vi "EXPT_IMGCAP.vi"(0 "Refnums":T1, 1 "Number of wavelengths":u16(ring) items=["1", "2", "3", "4", "5", "6"], 5 "Saved positions":dbl[][](array[numeric]), 9 "Filter array":dbl[](array[numeric]), 11 "Error in":errorcluster, 12 "Img data":refnum<queue>, 13 "State queue cam":refnum<queue>) -> (4 "Avg intensity":T2(array[cluster]), 6 "Number of positions":i32, 8 "XYZpos":cluster{dbl, dbl, dbl}, 15 "error out":errorcluster)   [LabVIEW 2018]
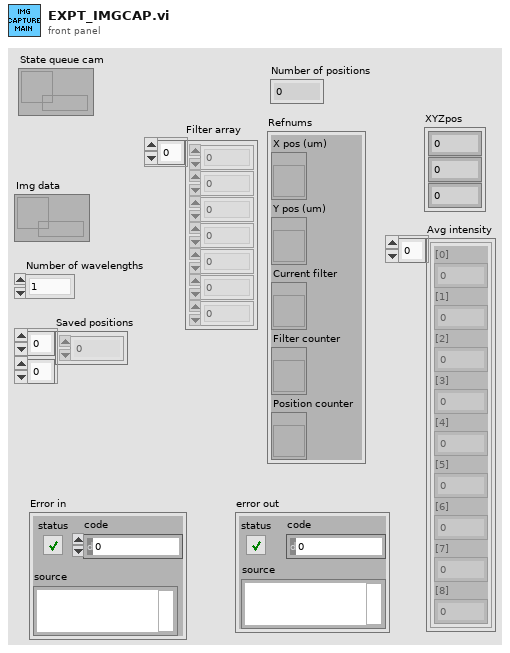
[diagram p1: front panel]
types:
  T1 = cluster{"X pos (um)":refnum<vi>, "Y pos (um)":refnum<vi>, "Current filter":refnum<vi>, "Filter counter":refnum<vi>, "Position counter":refnum<vi>}
  T2 = cluster{"[0]":dbl, "[1]":dbl, "[2]":dbl, "[3]":dbl, "[4]":dbl, "[5]":dbl, "[6]":dbl, "[7]":dbl, "[8]":dbl}[]
  T3 = enum16{"Wait", "Shutdown", "Start camera", "Shutdown camera", "Acquire", "Video ON", "Acquire series"}
  T4 = cluster{"[0]":dbl, "[1]":dbl, "[2]":dbl, "[3]":dbl, "[4]":dbl, "[5]":dbl, "[6]":dbl, "[7]":dbl, "[8]":dbl}
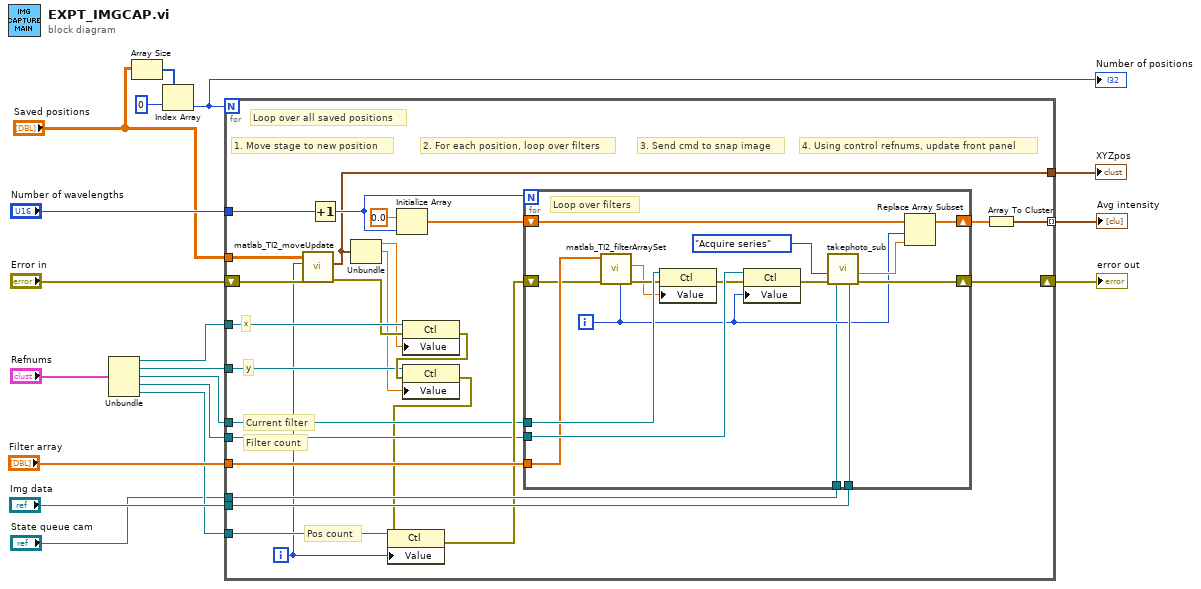
[diagram p0: block diagram]
diagram:
  n1 = Unbundle("Refnums") -> ("X pos (um)"=w12:refnum<vi>, "Y pos (um)"=w10:refnum<vi>, "Current filter"=w9:refnum<vi>, "Filter counter"=w8:refnum<vi>, "Position counter"=w7:refnum<vi>)
  n2 = Array Size(array="Saved positions") -> (size(s)=w4:i32[])
  n3 = Index Array(array=w4, index=0) -> (element=w1:i32)
  "Number of positions" <- w1
  n4 = for {
    N: w1 -> [_]
    tunnel: "Saved positions" -> [w21]
    shift-right: [w43] -> w16
    shift-left: "Error in" -> [w26]
    tunnel: "State queue cam" -> [w42]
    tunnel: [w24] -> w6
    tunnel: "Img data" -> [w39]
    tunnel: [w36] -> w17 mode=indexing
    tunnel: "Number of wavelengths" -> [w35]
    tunnel: w7 -> [w34]
    tunnel: "Filter array" -> [w33]
    tunnel: w12 -> [w30]
    tunnel: w10 -> [w27]
    tunnel: w9 -> [w29]
    tunnel: w8 -> [w28]
    i -> [w20]
    # "4. Using control refnums, update front panel"
    # "3. Send cmd to snap image"
    # "2. For each position, loop over filters"
    # "1. Move stage to new position"
    # "Filter count"
    # "Current filter"
    # "y"
    # "x"
    # "Pos count"
    # "Loop over all saved positions"
    n5 = call "matlab_TI2_moveUpdate.vi"("error in (no error)"=w26, "Position counter"=w20, "Saved positions"=w21) -> ("error out"=w25:errorcluster, "XYZpos"=w24:cluster{dbl, dbl, dbl})  [unwired: 7 in]
    n6 = Increment(x=w35) -> (x+1=w40:u16)
    n7 = Unbundle(w24) -> (w23:dbl, w22:dbl)  [unwired: 1 out]
    n8 = Initialize Array(0.0 ("element"), w40) -> (w38:dbl[])
    n9 = property class="Ctl"(reference=w30, error in=w25, "Value"=w23) -> (error out=w32:errorcluster)  [unwired: 1 out]
    n10 = property class="Ctl"(reference=w27, error in=w32, "Value"=w22) -> (error out=w19:errorcluster)  [unwired: 1 out]
    n11 = property class="Ctl"(reference=w34, error in=w19, "Value"=w20) -> (error out=w31:errorcluster)  [unwired: 1 out]
    n12 = for {
      N: w40 -> [_]
      shift-right: [w56] -> w43
      shift-left: w31 -> [w48]
      tunnel: w42 -> [w44]
      tunnel: w39 -> [w57]
      shift-right: [w58] -> w37
      shift-left: w38 -> [w59]
      tunnel: w29 -> [w54]
      tunnel: w28 -> [w53]
      tunnel: w33 -> [w50]
      i -> [w49]
      # "Loop over filters"
      n13 = call "matlab_TI2_filterArraySet.vi"("error in"=w48, "Filter index"=w49, "Filter array"=w50) -> ("error out"=w47:errorcluster, "Current filter"=w46:dbl)  [unwired: 7 in]
      n14 = property class="Ctl"(reference=w54, error in=w47, "Value"=w46) -> (error out=w52:errorcluster)  [unwired: 1 out]
      n15 = property class="Ctl"(reference=w53, error in=w52, "Value"=w49) -> (error out=w51:errorcluster)  [unwired: 1 out]
      n16 = call "takephoto_sub.vi"("error in (no error)"=w51, "States Cam"=T3."Acquire series", "Img data"=w57, "Queue in"=w44) -> ("error out"=w56:errorcluster, "Average intensity"=w55:dbl)  [unwired: 6 in]
      n17 = Replace Array Subset(array=w59, new element=w55, index=w49) -> (w58:dbl[])
    }
    n18 = Array To Cluster(array=w37) -> (cluster=w36:T4)
  }
  "error out" <- w16
  "Avg intensity" <- w17
  "XYZpos" <- w6
